vi "deleteSecKey.vi"(0 "HGF_GPG in":refnum<class "HGF_GPG.lvclass">, 1 "options file":path, 2 "keyringfile":path, 3 "Sec keyringfile":path, 5 "error in (no error)":errorcluster, 6 "key-id":string, 8 "Trust DB":path) -> (10 "dup Trust DB":path, 11 "success":bool, 14 "HGF_GPG out":refnum<class "HGF_GPG.lvclass">, 15 "dup options file":path, 16 "dup keyringfile":path, 17 "dup Sec keyringfile":path, 19 "error out":errorcluster)   [LabVIEW 2012, in "HGF_GPG.lvlib" / "HGF_GPG.lvclass"]
doc: "deletes the secret key with <b>key-id</b>"
uses:
  HGF_GPG.lvclass
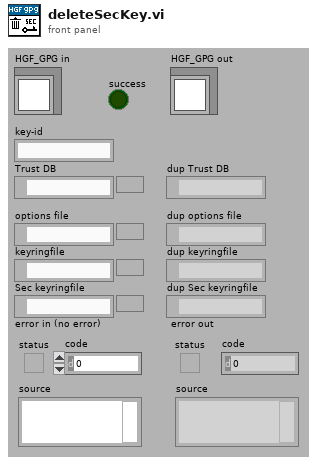
[diagram p1: front panel]
types:
  T1 = enum16{"list keys", "export", "import", "delete"}
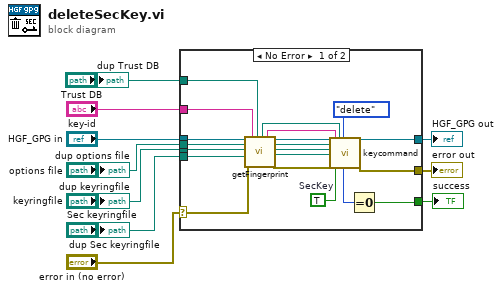
[diagram p0: block diagram]
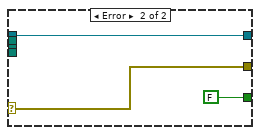
[diagram p2: hidden frame]
diagram:
  n1 = case shown="No Error" "error in (no error)" {
    selector: "error in (no error)" -> [w26 w33]
    tunnel: [w25 w33] -> w9
    tunnel: [w28 w32] -> w7
    tunnel: "HGF_GPG in" -> [w30 w32]
    tunnel: "key-id" -> [w17 _]
    tunnel: [w24 FALSE] -> w5
    tunnel: "keyringfile" -> [w19 _]
    tunnel: "options file" -> [w18 _]
    tunnel: "Sec keyringfile" -> [w15 _]
    tunnel: "Trust DB" -> [w13 _]
    frame No Error {
      w23 = TRUE  # SecKey
      n2 = call-dynamic "getFingerprint.vi"("HGF_GPG in"=w30, "options file"=w18, "keyringfile"=w19, "Sec keyringfile"=w15, "error in (no error)"=w26, "key-id"=w17, "Trust DB"=w13) -> ("dup Trust DB"=w12:path, "fingerprint"=w16:string, "dup HGF_GPG"=w29:refnum<class "HGF_GPG.lvclass">, "dup options file"=w20:path, "dup keyringfile"=w21:path, "dup Sec keyringfile"=w14:path, "error out"=w27:errorcluster)  [unwired: 6 out]
      n3 = call-dynamic "keycommand.vi"("HGF_GPG in"=w29, "options file"=w20, "keyringfile"=w21, "Sec keyringfile"=w14, "error in (no error)"=w27, "key-id"=w16, "SecKey (f)"=w23, "Trust DB"=w12, "Enum"=T1."delete") -> ("return code"=w22:i32, "HGF_GPG out"=w28:refnum<class "HGF_GPG.lvclass">, "error out"=w25:errorcluster)  [unwired: 2 in, 14 out]
      n4 = Equal To 0?(x=w22) -> (x = 0?=w24:bool)
    }
    frame Error {
    }
  }
  "error out" <- w9
  "HGF_GPG out" <- w7
  "success" <- w5
  "dup options file" <- "options file"
  "dup keyringfile" <- "keyringfile"
  "dup Sec keyringfile" <- "Sec keyringfile"
  "dup Trust DB" <- "Trust DB"
